vi "Pause timing.vi"(8 "error in (no error)":errorcluster, 10 "Station":T1, 11 "Car Wash Controller in":refnum<class "Car Wash Controller.lvclass">) -> (0 "error out":errorcluster, 3 "Car Wash Controller out":refnum<class "Car Wash Controller.lvclass">)   [LabVIEW 2019, in "Car Wash Controller.lvlib" / "Car Wash Controller.lvclass"]
uses:
  Car Wash Controller.lvclass
  Vehicle Position Simulation Actor/Car Wash Controller/Station -Enum.ctl
  Car Wash Controller.lvclass/Car Wash Controller.ctl
  Vehicle Position Simulation Actor/Car Wash Controller/Vehicle Position Simulation Actor.lvclass
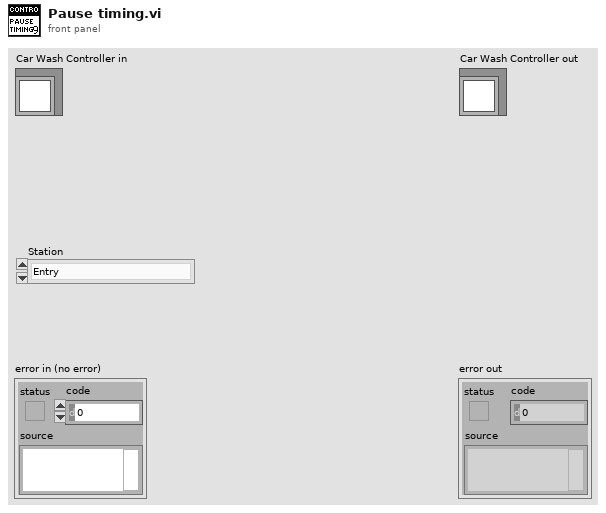
[diagram p1: front panel]
types:
  T1 = typedef "Vehicle Position Sinmulation Actor.lvlib/Vehicle Position Simulation Actor.lvclass/Station -Enum.ctl" = enum16{"Entry", "Station1", "Station2", "Station3", "Exit"}
  T2 = typedef "Car Wash Controller.lvlib/Car Wash Controller.lvclass/Staion_Wash Step_timing List.ctl" = string[][]
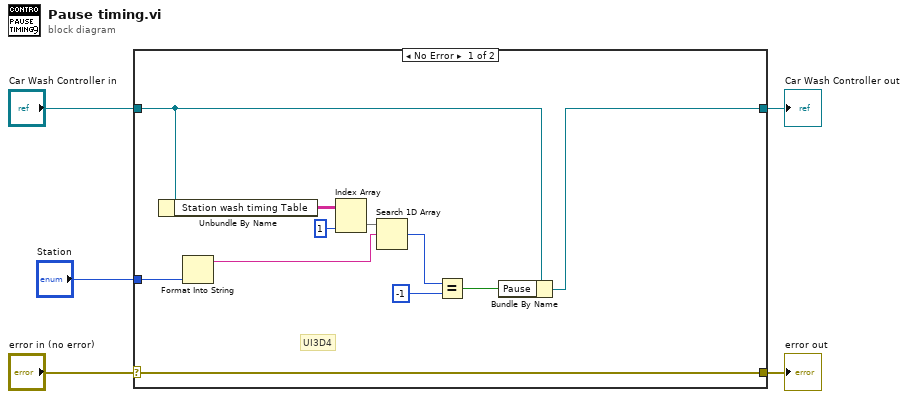
[diagram p0: block diagram]
diagram:
  n1 = case shown="No Error" "error in (no error)" {
    selector: "error in (no error)" -> [w16 w18]
    tunnel: [w16 w18] -> w4
    tunnel: [w7 w17] -> w2
    tunnel: "Car Wash Controller in" -> [w15 w17]
    tunnel: "Station" -> [w11 _]
    frame No Error {
      # "UI3D4"
      n2 = Unbundle By Name(w15) -> ("Station wash timing Table"=w14:T2)
      n3 = Format Into String(w11) -> (resulting string=w10:string)  [unwired: 3 in, 1 out]
      n4 = Index Array(array=w14, index (col)=1 ("disabled index (col)")) -> (element=w13:string[])  [unwired: 1 in]
      n5 = Search 1D Array(1D array=w13, element=w10) -> (index of element=w8:i32)  [unwired: 1 in]
      n6 = Equal?(x=w8, y=-1) -> (x = y?=w6:bool)
      n7 = Bundle By Name(cluster=w15, "Pause"=w6) -> (w7:refnum<class "Car Wash Controller.lvclass">)
    }
    frame Error {
    }
  }
  "error out" <- w4
  "Car Wash Controller out" <- w2
